vi "Joystick 2 Trigger.vi"() -> ()   [LabVIEW 2017]
panel:
  out "Simulated Joystick 2 Trigger":bool
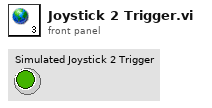
[diagram p1: front panel]
diagram:
